vi "Generate Waveform.vi"(0 "SV Discrete Sweep in":refnum<class "SV Discrete Sweep.lvclass">, 5 "template waveform":waveform(dbl), 9 "samples":i32, 11 "error in (no error)":errorcluster) -> (4 "SV Discrete Sweep out":refnum<class "SV Discrete Sweep.lvclass">, 6 "sine waveform":waveform(dbl), 10 "samples":i32, 15 "error out":errorcluster)   [LabVIEW 2017, in "SV Discrete Sweep.lvclass"]
uses:
  <vilib>/addons/_NISVFA/_Generation/Signal Generation/SV Discrete Sweep/SV Discrete Sweep.lvclass
  C:/Program Files (x86)/National Instruments/LabVIEW 2017/vi.lib/addons/_NISVFA/_Generation/Signal Generation/SV Signal/SV Signal.lvclass
  C:/Program Files (x86)/National Instruments/LabVIEW 2017/vi.lib/addons/_NISVFA/_Generation/Signal Generation/SV Function/SV Function.lvclass
  <vilib>/addons/_NISVFA/_Generation/Signal Generation/SV Discrete Sweep/SV Discrete Sweep.lvclass/SV Discrete Sweep.ctl
  <vilib>/addons/_NISVFA/_Generation/Signal Generation/SV Signal/sv_Signal State Attribute.ctl
  <vilib>/addons/_NISVFA/_Generation/Signal Generation/SV Signal/Read Sample Rate.vi
  <vilib>/Analysis/NI_AALBase.lvlib
  <vilib>/addons/_NISVFA/_Generation/Signal Generation/SV Function/SV Function.lvclass
  <vilib>/addons/_NISVFA/_Generation/Signal Generation/SV Signal/SV Signal.lvclass
  <vilib>/measure/NI_MABase.lvlib
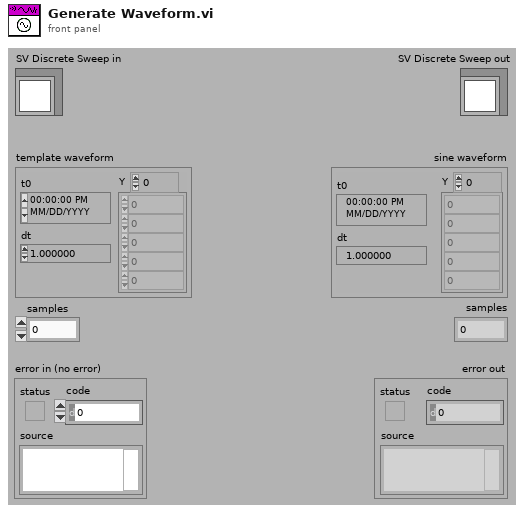
[diagram p1: front panel]
types:
  T1 = typedef "SV Signal.lvclass/sv_Signal State Attribute.ctl" = string
  T2 = typedef "SV Signal.lvclass/sv_System Timing Model.ctl" = i64
  T3 = typedef "SV Signal.lvclass/sv_Generation State.ctl" = enum16{"Idle", "Ramp Up", "Pre-Measurement Settling", "Measurement", "Post-Measurement Settling", "Discrete Sweep Transition", "Ramp Down", "Update"}
  T4 = cluster{"system timing model":T2, "state":cluster{"RESET":bool, "generator timestamp":timestamp, "elapsed seconds":dbl, "elapsed samples":u64, "generation state":T3, "time offset at state":dbl, "samples generated at state":u64, "signal state":variant}, "duration of state":dbl, "samples remaining at state":i32}
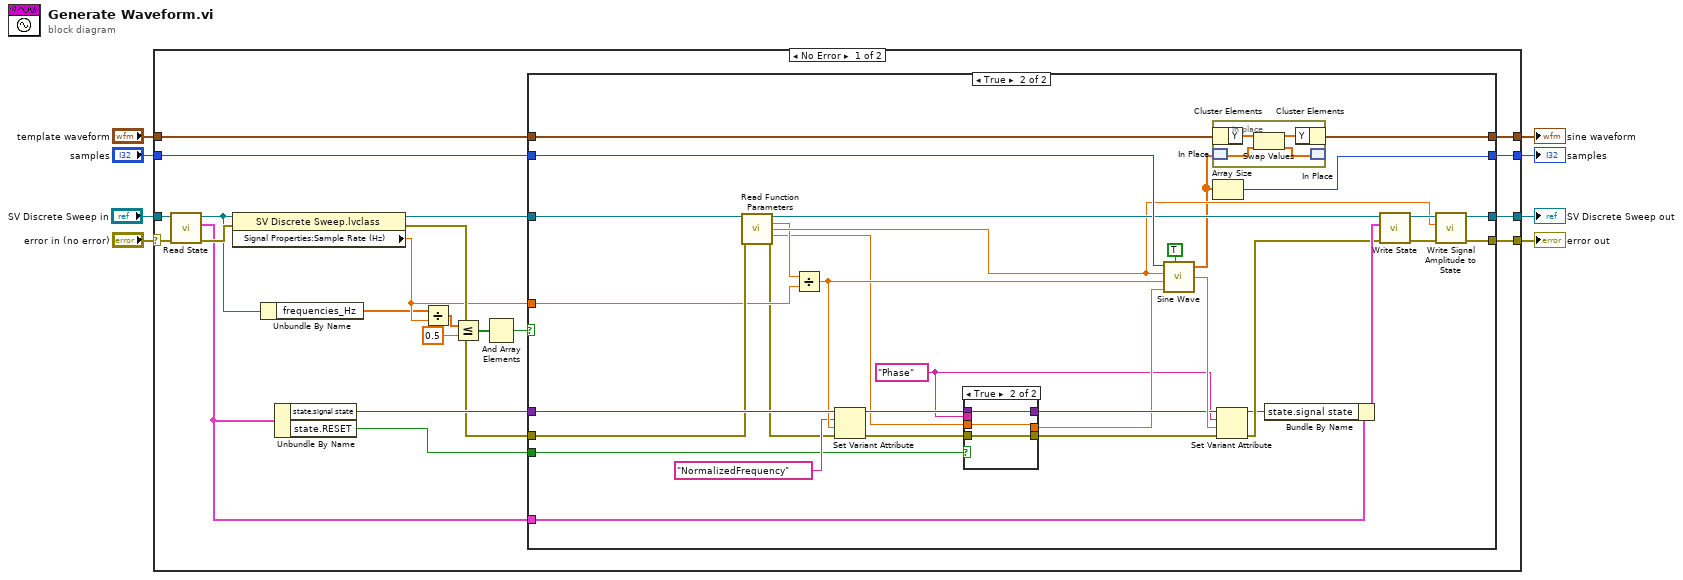
[diagram p0: block diagram]
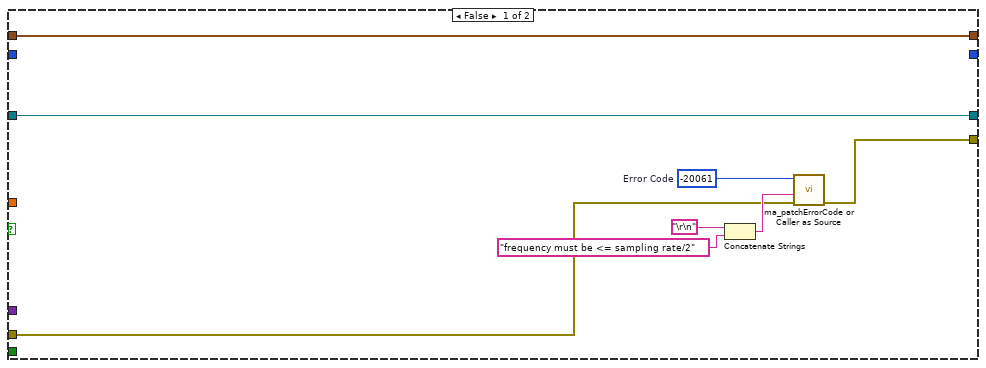
[diagram p2: hidden frame]
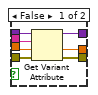
[diagram p3: hidden frame]
diagram:
  n1 = case shown="No Error" "error in (no error)" {
    selector: "error in (no error)" -> [w27 w87]
    tunnel: [w18 w87] -> w7
    tunnel: [w17 w86] -> w5
    tunnel: "SV Discrete Sweep in" -> [w22 w86]
    tunnel: "template waveform" -> [w29 w85]
    tunnel: [w28 w85] -> w3
    tunnel: "samples" -> [w20 _]
    tunnel: [w19 _] -> w1
    frame No Error {
      n2 = call <vilib>:"Read State.vi"("error in (no error)"=w27, "signal configuration"=w22) -> ("error out"=w25:errorcluster, "generator state"=w21:T4, "signal configuration"=w16:refnum<class "SV Discrete Sweep.lvclass">)  [unwired: 7 in]
      n3 = property class="SV Discrete Sweep.lvclass"(reference=w16, error in=w25) -> (reference out=w23:refnum<class "SV Discrete Sweep.lvclass">, error out=w24:errorcluster, "Signal Properties:Sample Rate (Hz)"=w13:dbl)
      n4 = Unbundle By Name(w16) -> ("frequencies_Hz"=w12:dbl[])
      n5 = Unbundle By Name(w21) -> ("state.signal state"=w26:variant, "state.RESET"=w9:bool)
      n6 = Divide(x=w12, y=w13) -> (x/y=w15:dbl[])
      n7 = Less Or Equal?(x=w15, y=0.5) -> (x <= y?=w11:bool[])
      n8 = And Array Elements(Boolean array=w11) -> (logical AND=w10:bool)
      n9 = case shown="True" w10 {
        tunnel: w29 -> [w37 w70]
        tunnel: [w37 w69] -> w28
        tunnel: w9 -> [_ w38]
        tunnel: w26 -> [_ w68]
        tunnel: w24 -> [w31 w67]
        tunnel: w23 -> [w36 w66]
        tunnel: w21 -> [_ w65]
        tunnel: w13 -> [_ w64]
        tunnel: w20 -> [_ w63]
        tunnel: [_ w62] -> w19
        tunnel: [w30 w54] -> w18
        tunnel: [w36 w55] -> w17
        frame False {
          w32 = -20061  # Error Code
          n10 = Concatenate Strings("\r\n", "frequency must be <= sampling rate/2" ("freq error message")) -> (w35:string)
          n11 = call <vilib>:"ma_patchErrorCode or Caller as Source.vi"("error in (no error)"=w31, "string to append to source"=w35, "error code"=w32) -> ("error out"=w30:errorcluster)  [unwired: 8 in]
        }
        frame True {
          w39 = T1 "Phase" ("name")
          n12 = call <vilib>:"Read Function Parameters.vi"("signal configuration"=w66, "error in (no error)"=w67) -> ("signal configuration"=w60:refnum<class "SV Discrete Sweep.lvclass">, "frequency_Hz"=w44:dbl, "amplitude"=w56:dbl, "initial_phase_deg"=w40:dbl, "error out"=w43:errorcluster)  [unwired: 8 in, 1 out]
          n13 = Divide(x=w44, y=w64) -> (x/y=w47:dbl)
          n14 = Set Variant Attribute(Variant=w68, name=T1 "NormalizedFrequency", value=w47, error in=w43) -> (Variant out=w42:variant, error out=w41:errorcluster)  [unwired: 1 out]
          n15 = case shown="True" w38 {
            tunnel: [w77 w78] -> w51
            tunnel: [w76 w79] -> w50
            tunnel: [w75 w80] -> w49
            tunnel: w42 -> [w74 w79]
            tunnel: w41 -> [w73 w78]
            tunnel: w40 -> [w72 w80]
            tunnel: w39 -> [w71 _]
            frame False {
              n16 = Get Variant Attribute(Variant=w74, name=w71, default value (empty Variant)=w72, error in=w73) -> (duplicate Variant=w76:variant, value=w75:dbl, error out=w77:errorcluster)  [unwired: 1 out]
            }
            frame True {
            }
          }
          n17 = call <vilib>:"Sine Wave.vi"("samples"=w63, "amplitude"=w56, "frequency"=w47, "phase in"=w49, "reset phase"=TRUE) -> ("sine wave"=w48:dbl[], "phase out"=w52:dbl)  [unwired: 1 out]
          n18 = in-place {
            n19 = in-place-cluster #1(w70) -> ("Y"=w84:dbl[])
            n20 = in-place-match #2(w48) -> (w82:dbl[])
            n21 = Swap Values(12:w84, 14:w82) -> (1:w83:dbl[], 3:w81:dbl[])  [unwired: 1 in]
            n22 = in-place-cluster #1("Y"=w83) -> (w69:waveform(dbl))
            n23 = in-place-match #2(w81) -> ()  [unwired: 1 out]
          }
          n24 = Array Size(array=w48) -> (size(s)=w62:i32)
          n25 = Set Variant Attribute(Variant=w50, name=w39, value=w52, error in=w51) -> (Variant out=w46:variant, error out=w58:errorcluster)  [unwired: 1 out]
          n26 = Bundle By Name(cluster=w65, "state.signal state"=w46) -> (w59:T4)
          n27 = call <vilib>:"Write State.vi"("error in (no error)"=w58, "generator state"=w59, "signal configuration"=w60) -> ("error out"=w61:errorcluster, "signal configuration"=w57:refnum<class "SV Discrete Sweep.lvclass">)  [unwired: 7 in]
          n28 = call <vilib>:"Write Signal Amplitude to State.vi"("error in (no error)"=w61, "amplitude"=w56, "SV Signal in"=w57) -> ("error out"=w54:errorcluster, "SV Signal out"=w55:refnum<class "SV Discrete Sweep.lvclass">)  [unwired: 7 in]
        }
      }
    }
    frame Error {
    }
  }
  "error out" <- w7
  "SV Discrete Sweep out" <- w5
  "sine waveform" <- w3
  "samples" <- w1
